vi "Fan&Temperature.vi"() -> ()   [LabVIEW 2011]
uses:
  Global/Globalclient.vi
panel:
  in  "stop":bool
  in  "Alarm":bool
  in  "风扇 4":string
  out "Ring 4":u16(ring)
  in  "风扇 3":string
  out "Ring 3":u16(ring)
  in  "风扇 2":string
  out "Ring 2":u16(ring)
  in  "风扇 1":string
  out "Ring 1":u16(ring)
  out "温度 8":dbl(slide)=50.0 scale=0.0..100.0 scale format="%0.1f"
  out "温度 7":dbl(slide)=50.0 scale=0.0..100.0 scale format="%0.1f"
  out "温度 6":dbl(slide)=50.0 scale=0.0..100.0 scale format="%0.1f"
  out "温度 5":dbl(slide)=50.0 scale=0.0..100.0 scale format="%0.1f"
  out "温度 4":dbl(slide)=50.0 scale=0.0..100.0 scale format="%0.1f"
  out "温度 3":dbl(slide)=50.0 scale=0.0..100.0 scale format="%0.1f"
  out "温度 2":dbl(slide)=50.0 scale=0.0..100.0 scale format="%0.1f"
  out "温度 1":dbl(slide)=50.0 scale=0.0..100.0 scale format="%0.1f"
  in  "机箱":T1(tab)
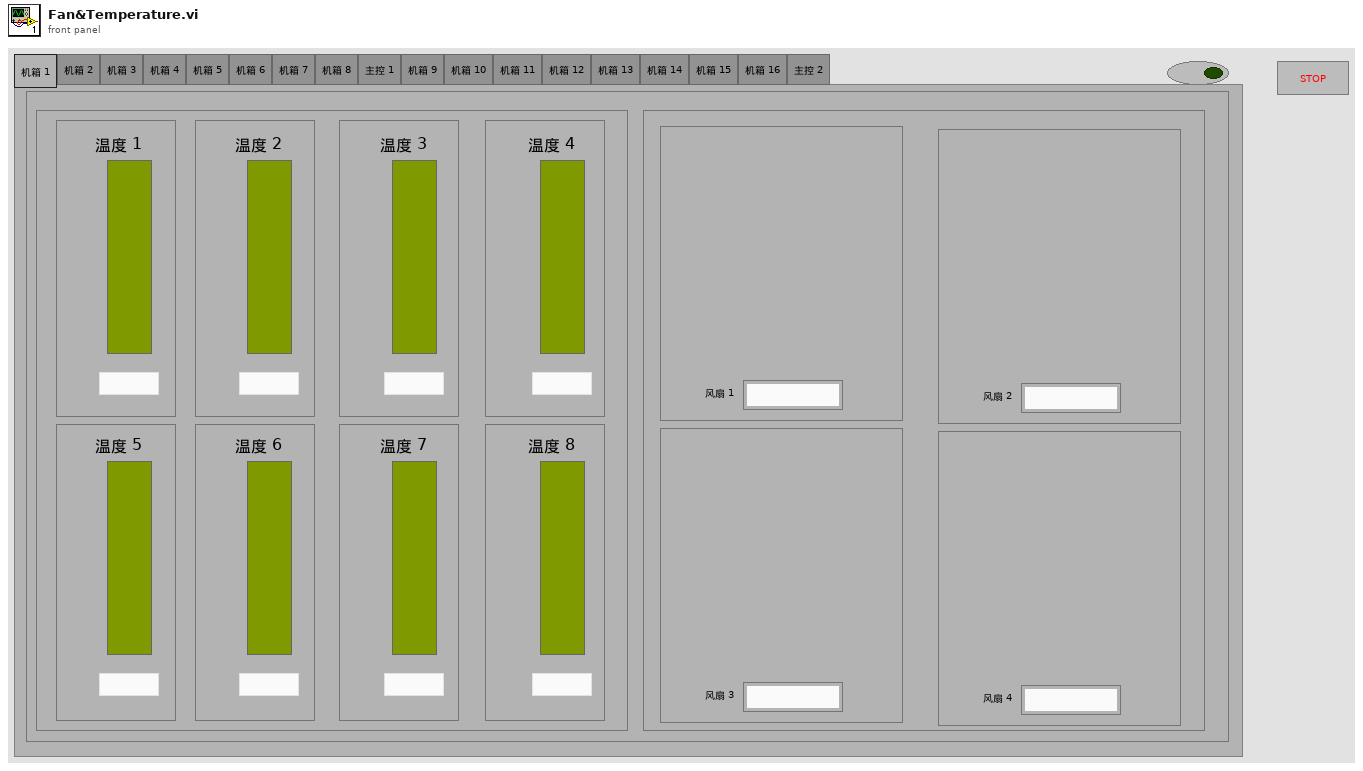
[diagram p1: front panel]
types:
  T1 = enum32{"机箱 1", "机箱 2", "机箱 3", "机箱 4", "机箱 5", "机箱 6", "机箱 7", "机箱 8", "主控 1", "机箱 9", "机箱 10", "机箱 11", "机箱 12", "机箱 13", "机箱 14", "机箱 15", "机箱 16", "主控 2"}
  T2 = enum16{"Standard", "Buffered", "CRLF", "Immediate"}
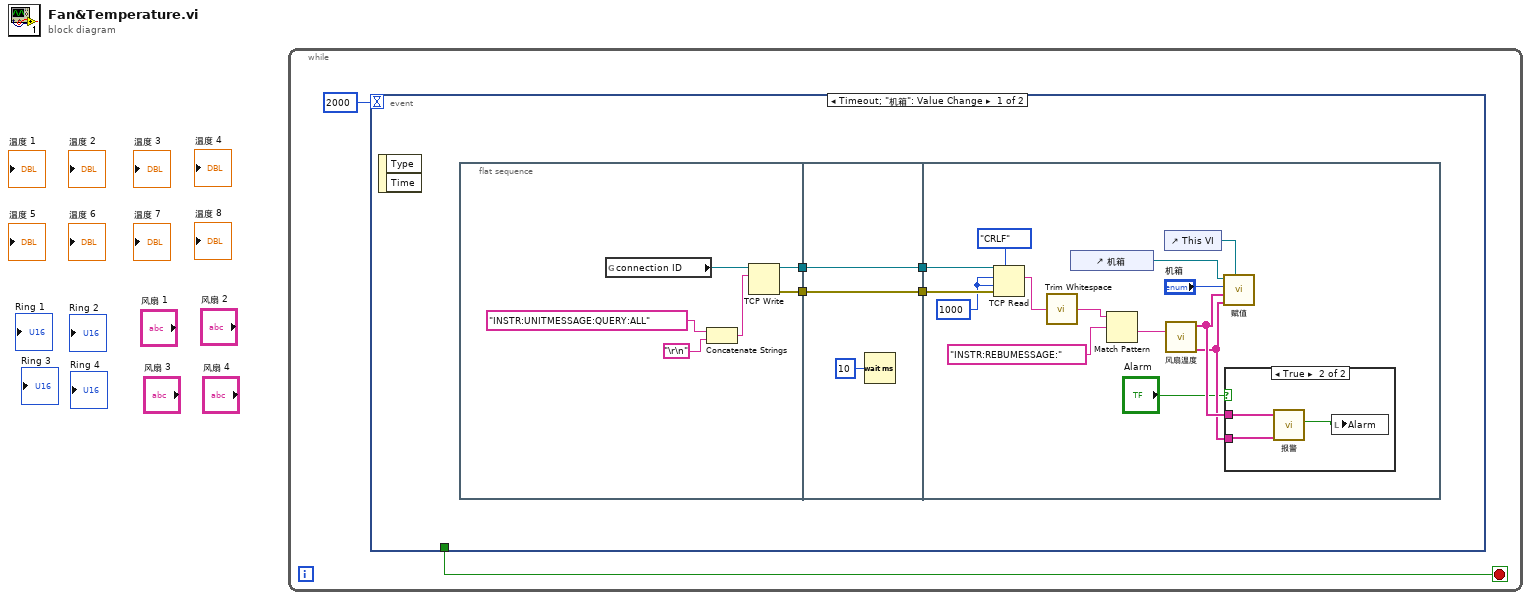
[diagram p0: block diagram]
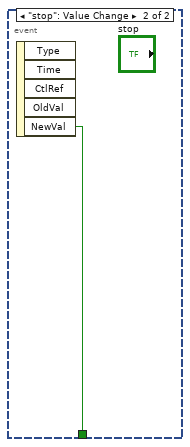
[diagram p3: hidden frame]
diagram:
  n1 = while {
    stop <- w1 stop-if-true
    n2 = event shown="[0] Timeout;  \"机箱\": Value Change" {
      selector: _ -> [_ _]
      dyn-events: _ -> [_ _]
      timeout: 2000 -> [_ _]
      tunnel: [_ w33] -> w1
      event Timeout; "机箱": Value Change {
        n3 = event-data() -> ()  [unwired: 1 in, 2 out]
        n4 = flat-sequence {
          tunnel: [w9] -> w6
          tunnel: [w8] -> w5
          tunnel: [w15] -> w4
          tunnel: w6 -> [w15]
          tunnel: [w14] -> w3
          tunnel: w5 -> [w14]
          tunnel: w4 -> [w29]
          tunnel: w3 -> [w28]
          frame #0 {
            n5 = global read "Globalclient.vi" "connection ID"() -> (w12:refnum<k5>)
            n6 = Concatenate Strings("INSTR:UNITMESSAGE:QUERY:ALL", "\r\n") -> (w10:string)
            n7 = TCP Write(connection ID=w12, data in=w10) -> (connection ID out=w9:refnum<k5>, error out=w8:errorcluster)  [unwired: 2 in, 1 out]
          }
          frame #1 {
            n8 = Wait (ms)(milliseconds to wait=u32 10) -> ()  [unwired: 1 out]
          }
          frame #2 {
            w27 = u32 1000 ("milliseconds to wait")
            n9 = TCP Read(connection ID=w29, bytes to read=w27, error in (no error)=w28, 7:T2."CRLF" ("mode (standard)"), 9:w27) -> (data out=w25:string)  [unwired: 2 out]
            n10 = call <vilib>:"Trim Whitespace.vi"("string"=w25) -> ("trimmed string"=w24:string)  [unwired: 1 in]
            n11 = control-ref of="机箱"() -> (w20:refnum<vi>)
            n12 = Match Pattern(string=w24, regular expression="INSTR:REBUMESSAGE:") -> (after substring=w22:string)  [unwired: 1 in, 3 out]
            n13 = control-ref of="This VI"() -> (w19:refnum<vi>)
            n14 = call "风扇温度.vi"("order"=w22) -> ("temp"=w17:string[], "fengshan"=w18:string[])  [unwired: 9 in]
            n15 = call "赋值.vi"("This VI"=w19, "temp"=w17, "fengshan"=w18, "机箱index"="机箱", "主控选项卡"=w20) -> ()  [unwired: 7 in]
            n16 = case shown="True" "Alarm" {
              tunnel: w18 -> [_ w32]
              tunnel: w17 -> [_ w31]
              frame False {
              }
              frame True {
                n17 = call "报警.vi"("temp"=w31, "fengshan"=w32) -> ("ALARM"=w30:bool)  [unwired: 9 in]
                n18 = local write "Alarm"(w30) -> ()
              }
            }
          }
        }
      }
      event "stop": Value Change {
        n19 = event-data() -> ("NewVal"=w33:bool)  [unwired: 1 in, 4 out]
      }
    }
  }
